vi "reset_state.vi"(0 "MoAgSy_AgentBase in":refnum<class "MoAgSy_AgentBase.lvclass">, 5 "error in (no error)":errorcluster) -> (14 "MoAgSy_AgentBase out":refnum<class "MoAgSy_AgentBase.lvclass">, 19 "error out":errorcluster)   [LabVIEW 2009, in "MoAgSy_Base.lvlib" / "MoAgSy_AgentBase.lvclass"]
uses:
  MoAgSy_AgentBase.lvclass
  MoAgSy_AgentBase.lvclass/MoAgSy_AgentBase.ctl
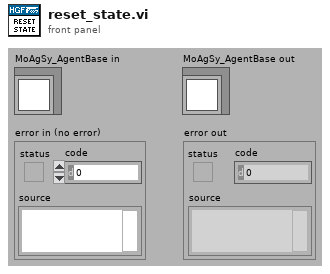
[diagram p1: front panel]
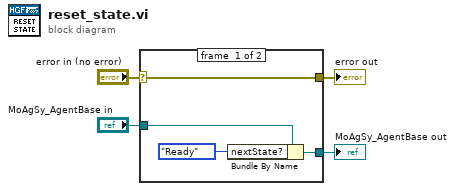
[diagram p0: block diagram]
diagram:
  n1 = case shown="No Error" "error in (no error)" {
    selector: "error in (no error)" -> [w7 w10]
    tunnel: [w7 w10] -> w3
    tunnel: [w6 w9] -> w1
    tunnel: "MoAgSy_AgentBase in" -> [w8 w9]
    frame #0 {
      n2 = Bundle By Name(cluster=w8, "nextState?"=enum16{"Ready", "stop", "travel"}."Ready") -> (w6:refnum<class "MoAgSy_AgentBase.lvclass">)
    }
    frame #1 {
    }
  }
  "error out" <- w3
  "MoAgSy_AgentBase out" <- w1
